vi "Find by Path Test.vi"() -> ()   [LabVIEW 2017]
uses:
  String Subset.vi
  Parsing/Parse Full Path or Item Name.vi
  Offset/Find Item Locations by Path.vi
  <vilib>/addons/_JKI Toolkits/Caraya/classes/Test/Test.lvclass
  <vilib>/addons/_JKI Toolkits/Caraya/classes/Assert/Assert.lvclass
  JSONtext.lvlib
panel:
  out "Array":string[](array[string])
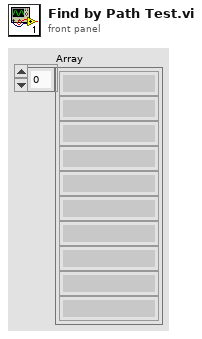
[diagram p1: front panel]
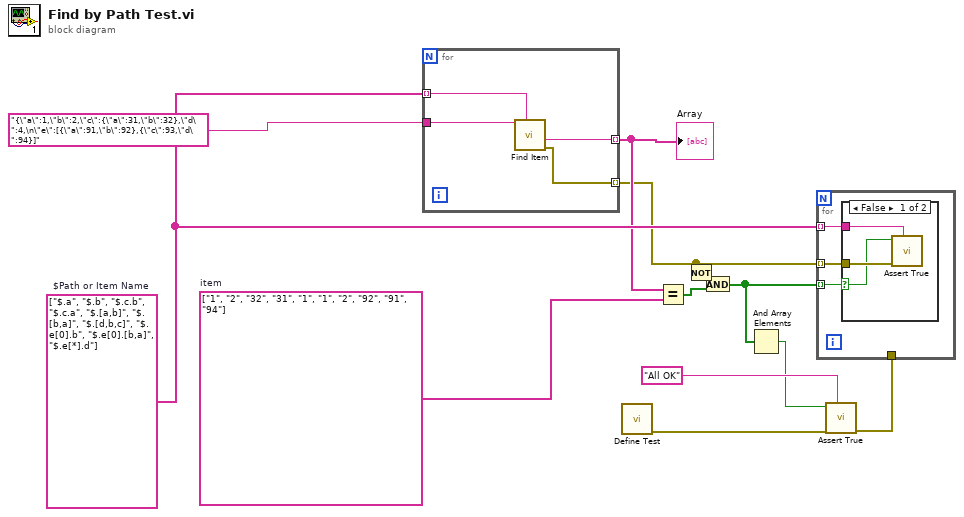
[diagram p0: block diagram]
diagram:
  w1 = string[] ["1", "2", "32", "31", "1", "1", "2", "92", "91", "94"]  # item
  w11 = string[] ["$.a", "$.b", "$.c.b", "$.c.a", "$.[a,b]", "$.[b,a]", "$.[d,b,c]", "$.e[0].b", "$.e[0].[b,a]", "$.e[*].d"]  # $Path or Item Name
  n1 = for {
    tunnel: "{\"a\":1,\"b\":2,\"c\":{\"a\":31,\"b\":32},\"d\":4,\n\"e\":[{\"a\":91,\"b\":92},{\"c\":93,\"d\":94}]" -> [w16]
    tunnel: w11 -> [w15] mode=indexing
    tunnel: [w14] -> w8 mode=indexing
    tunnel: [w13] -> w6 mode=indexing
    n2 = call "Find Item.vi"("$Path or Item Name"=w15, "JSON"=w16) -> ("error out"=w13:errorcluster, "<JSON>"=w14:string)  [unwired: 6 in, 2 out]
  }
  "Array" <- w8
  n3 = call <vilib>:"Define Test.vi"() -> ("error out"=w10:errorcluster)  [unwired: 11 in]
  n4 = Equal?(x=w8, y=w1) -> (x = y?=w7:bool[])
  n5 = Not(x=w6) -> (.not. x?=w5:bool[])
  n6 = And(x=w5, y=w7) -> (x .and. y?=w4:bool[])
  n7 = And Array Elements(Boolean array=w4) -> (logical AND=w3:bool)
  n8 = call <vilib>:"Assert True.vi"("Label"="All OK", "error in (no error)"=w10, "True?"=w3) -> ("error out"=w2:errorcluster)  [unwired: 8 in]
  n9 = for {
    tunnel: w11 -> [w19] mode=indexing
    tunnel: w6 -> [w18] mode=indexing
    tunnel: w4 -> [w17] mode=indexing
    tunnel: w2 -> [_]
    n10 = case shown="False" w17 {
      selector: w17 -> [w20 _]
      tunnel: w19 -> [w22 _]
      tunnel: w18 -> [w21 _]
      frame False {
        n11 = call <vilib>:"Assert True.vi"("Label"=w22, "error in (no error)"=w21, "True?"=w20) -> ()  [unwired: 8 in, 1 out]
      }
      frame True {
      }
    }
  }
